vi "Set exposure.vi"(8 "error in (no error)":errorcluster, 11 "DAQOrcaFlash in":refnum<class "DAQOrcaFlash.lvclass">) -> (0 "error out":errorcluster, 3 "DAQOrcaFlash out":refnum<class "DAQOrcaFlash.lvclass">)   [LabVIEW 2012, in "DAQOrcaFlash.lvclass"]
uses:
  DAQOrcaFlash.lvclass
  DAQOrcaFlash.lvclass/DAQOrcaFlash.ctl
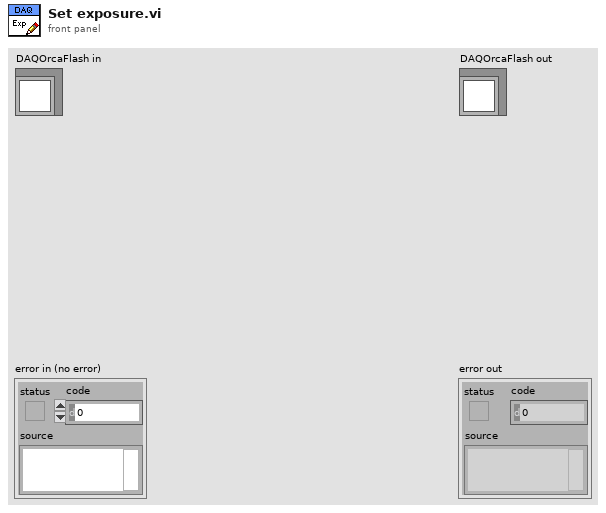
[diagram p1: front panel]
types:
  T1 = typedef "DAQOrcaFlash.lvclass/sensor_mode.ctl" = sgl
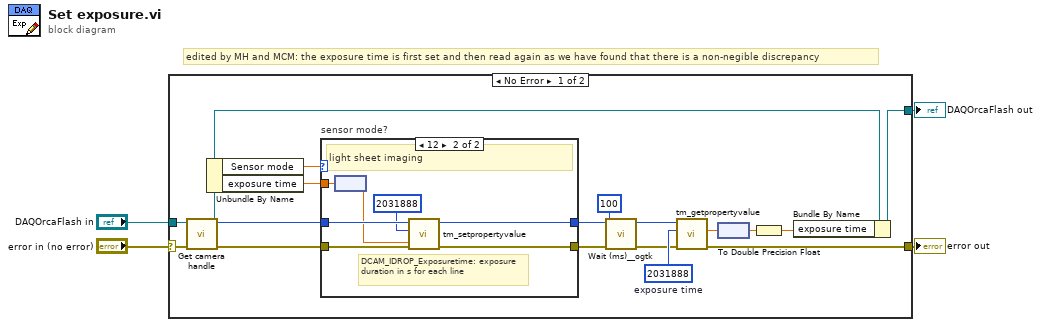
[diagram p0: block diagram]
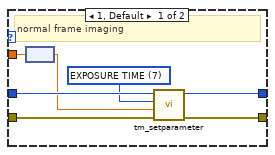
[diagram p2: hidden frame]
diagram:
  # "edited by MH and MCM: the exposure time is first set and then read again as we have found that there is a non-negible discrepancy"
  n1 = case shown="No Error" "error in (no error)" {
    selector: "error in (no error)" -> [w21 w37]
    tunnel: [w5 w37] -> w3
    tunnel: [w10 w36] -> w1
    tunnel: "DAQOrcaFlash in" -> [w17 w36]
    frame No Error {
      w16 = u32 2031888  # exposure time
      n2 = call "Get camera handle.vi"("error in (no error)"=w21, "DAQMH121119OrcaFlash in"=w17) -> ("error out"=w20:errorcluster, "cam handle"=w19:u32, "DAQMH121119OrcaFlash out"=w11:refnum<class "DAQOrcaFlash.lvclass">)  [unwired: 7 in]
      n3 = Unbundle By Name(w11) -> ("Sensor mode"=w8:T1, "exposure time"=w18:dbl[unit])
      n4 = case "sensor mode?" shown="12" w8 {
        tunnel: w20 -> [w28 w35]
        tunnel: w19 -> [w26 w34]
        tunnel: w18 -> [w24 w33]
        tunnel: [w27 w30] -> w12
        tunnel: [w22 w29] -> w15
        frame 1, Default {
          w25 = u32 7 items=["BINNING"=1, "BITS PER CHANNEL"=2, "ACTIVE VIEW INDEX"=3, "CCD MODE"=4, "SENSOR MODE"=5, "READOUT MODE"=6, "EXPOSURE TIME"=7, "CONTRAST GAIN"=8, "CONTRAST OFFSET"=9, "LIGHT MODE"=10, "SENSITIVITY"=11, "WHITE BALANCE"=12, "PHOTON IMAGING MODE"=13, "HIGH DYNAMIC RANGE MODE"=14, "TRIGGER SOURCE"=15, "TRIGGER ACTIVE"=16, "TRIGGER MODE"=17, "TRIGGER POLARITY"=18, "TRIGGER GLOBAL EXPOSURE"=19, "FIRST TRIGGER BEHAVIOR"=20, "TRIGGER TIMES"=21, "OUTPUT TRIGGER POLARITY"=22, "OUTPUT TRIGGER DELAY"=23, "OUTPUT TRIGGER PERIOD"=24, "TEMPERATURE"=25, "TEMPERATURE TARGET"=26, "SENSOR COOLER FAN"=27, "MECHANICAL SHUTTER"=28, "BACK FOCUS POSITION"=29, "FRAMEBUNDLE MODE"=30, "FRAMEBUNDLE NUMBER"=31, "LINEBUNDLE HEIGHT"=32, "TRIGGER CONNECTOR"=33, "IMAGE PIXEL TYPE"=34, "OUTPUT TRIGGER KIND"=35, "READOUT DIRECTION"=36] ("Parameter")
          # "normal frame imaging"
          n5 = node(w24) -> (w23:dbl)
          n6 = call <userlib>:"tm_setparameter.vi"("error in (no error)"=w28, "Value in"=w23, "Parameter"=w25, "Handle in"=w26) -> ("error out"=w27:errorcluster, "Handle out"=w22:u32)  [unwired: 6 in]
        }
        frame 12 {
          # "DCAM_IDROP_Exposuretime: exposure duration in s for each line"
          # "light sheet imaging"
          n7 = node(w33) -> (w32:dbl)
          n8 = call <userlib>:"tm_setpropertyvalue.vi"("error in (no error)"=w35, "Value in"=w32, "Property ID"=u32 2031888, "Handle in"=w34) -> ("error out"=w30:errorcluster, "Handle out"=w29:u32)  [unwired: 6 in]
        }
      }
      n9 = call <userlib>:"Wait (ms)__ogtk.vi"("error in (no error)"=w12, "milliseconds to wait"=u32 100) -> ("error out"=w13:errorcluster)  [unwired: 8 in, 1 out]
      n10 = call <userlib>:"tm_getpropertyvalue.vi"("error in (no error)"=w13, "Property ID"=w16, "Handle in"=w15) -> ("error out"=w5:errorcluster, "Value in"=w9:sgl)  [unwired: 6 in, 1 out]
      n11 = node(w9) -> (w7:sgl[unit])
      n12 = To Double Precision Float(number=w7) -> (double precision float=w6:dbl[unit])
      n13 = Bundle By Name(cluster=w11, "exposure time"=w6) -> (w10:refnum<class "DAQOrcaFlash.lvclass">)
    }
    frame Error {
    }
  }
  "error out" <- w3
  "DAQOrcaFlash out" <- w1
